vi "Enforce Set-Points.vi"(0 "Experimental Queue":T1) -> ()   [LabVIEW 2013]
uses:
  Runtime/Runtime Queue.ctl
  Runtime/Experimental Configuration.ctl
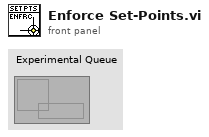
[diagram p1: front panel]
types:
  T1 = typedef "Runtime Queue.ctl" = refnum<queue>
  T2 = typedef "Experimental Configuration.ctl" = cluster{"Output Waveforms":waveform(dbl)[], "Output Channels":string, "Input Channels":string, "Post-Hook Occurence":refnum<k4>}
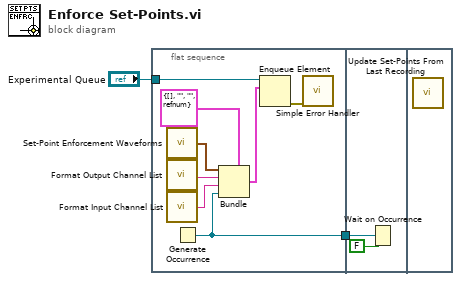
[diagram p0: block diagram]
diagram:
  n1 = flat-sequence {
    tunnel: [w8] -> w1
    tunnel: "Experimental Queue" -> [w10]
    tunnel: w1 -> [w12]
    frame #0 {
      n2 = call "Set-Point Enforcement Waveforms.vi"() -> ("Output Waveforms"=w6:waveform(dbl)[])
      n3 = call "Format Output Channel List.vi"() -> ("Output Channels"=w7:string)
      n4 = call "Format Input Channel List.vi"() -> ("Input Channels"=w5:string)
      n5 = Generate Occurrence() -> (w8:refnum<k4>)
      n6 = Bundle(cluster=T2 {"Output Waveforms"=[], "Output Channels"="", "Input Channels"="", "Post-Hook Occurence"=refnum} ("Experimental Configuration"), "Output Waveforms"=w6, "Output Channels"=w7, "Input Channels"=w5, "Post-Hook Occurence"=w8) -> (w3:T2)
      n7 = Enqueue Element(queue=w10, element=w3) -> (error out=w9:errorcluster)  [unwired: 2 in, 2 out]
      n8 = call <vilib>:"Simple Error Handler.vi"("error in (no error)"=w9) -> ()  [unwired: 4 in, 5 out]
    }
    frame #1 {
      n9 = Wait on Occurrence(1:FALSE ("ignore previous (T)"), 2:w12) -> ()  [unwired: 1 in, 1 out]
    }
    frame #2 {
      n10 = call "Update Set-Points From Last Recording.vi"() -> ()  [unwired: 1 in]
    }
  }
